vi "judge.vi"(1 "Cluster":T1) -> (0 "logical AND":bool)   [LabVIEW 2018]
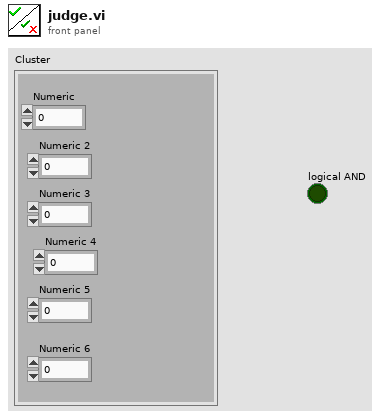
[diagram p1: front panel]
types:
  T1 = cluster{"Numeric":dbl, "Numeric 2":dbl, "Numeric 3":dbl, "Numeric 4":dbl, "Numeric 5":dbl, "Numeric 6":dbl}
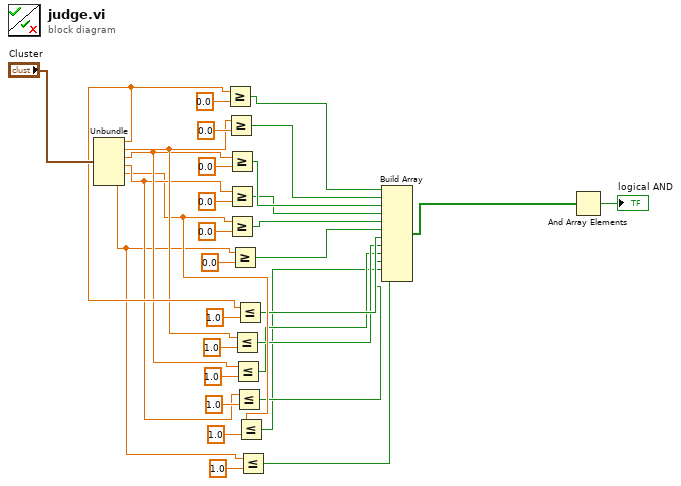
[diagram p0: block diagram]
diagram:
  n1 = Unbundle("Cluster") -> ("Numeric"=w12:dbl, "Numeric 2"=w11:dbl, "Numeric 3"=w10:dbl, "Numeric 4"=w9:dbl, "Numeric 5"=w8:dbl, "Numeric 6"=w7:dbl)
  n2 = Greater Or Equal?(x=w12, y=0.0) -> (x >= y?=w26:bool)
  n3 = Greater Or Equal?(x=w11, y=0.0) -> (x >= y?=w25:bool)
  n4 = Greater Or Equal?(x=w10, y=0.0) -> (x >= y?=w24:bool)
  n5 = Greater Or Equal?(x=w9, y=0.0) -> (x >= y?=w23:bool)
  n6 = Greater Or Equal?(x=w8, y=0.0) -> (x >= y?=w22:bool)
  n7 = Greater Or Equal?(x=w7, y=0.0) -> (x >= y?=w21:bool)
  n8 = Less Or Equal?(x=w11, y=1.0) -> (x <= y?=w5:bool)
  n9 = Less Or Equal?(x=w10, y=1.0) -> (x <= y?=w4:bool)
  n10 = Less Or Equal?(x=w9, y=1.0) -> (x <= y?=w3:bool)
  n11 = Less Or Equal?(x=w12, y=1.0) -> (x <= y?=w6:bool)
  n12 = Less Or Equal?(x=w8, y=1.0) -> (x <= y?=w2:bool)
  n13 = Less Or Equal?(x=w7, y=1.0) -> (x <= y?=w1:bool)
  n14 = Build Array(w26, w25, w24, w23, w22, w21, w6, w5, w4, w3, w2, w1) -> (w20:bool[])
  n15 = And Array Elements(Boolean array=w20) -> (logical AND=→"logical AND":bool)
